vi "PH_TKTDS-30xx.ProcCases.vi"(0 "i ref in":refnum<vi>, 1 "selector":string, 2 "Data":T1, 3 "call cluster":T2={"Object"="", "Selector"="", "CallType"=enum."synchronous", "Async Object"="", "Async Selector"="", "Data Descriptor"="", "Data"=[], "Error #"=0, "Expire"=0}, 5 "error in (no error)":errorcluster) -> (14 "i ref out":refnum<vi>, 17 "answer cluster":T2={"Object"="", "Selector"="", "CallType"=enum."synchronous", "Async Object"="", "Async Selector"="", "Data Descriptor"="", "Data"=[], "Error #"=0, "Expire"=0}, 19 "error out":errorcluster)   [LabVIEW 2014, in "PH_TKTDS-30xx.lvlib"]
doc: "This method is called by a process from within the default case in the event loop. The methods of a class that are linked to events will be called from THIS method. Add your code here."
uses:
  PH_TKTDS-30xx.lvlib
  CS_Core/CSSystem/CoreDefs/CoreDefs.call_type.ctl
  CS_Core/BaseProcess/BaseProcess.descriptor string definition.ctl
  CS_Core/CSSystem/CoreDefs/CoreDefs.rawDataType.ctl
  PH_TKTDS-30xx.Channel Config.ctl
  PH_TKTDS-30xx.Acquisition Config.ctl
  PH_TKTDS-30xx.Trigger Config.ctl
  PH_TKTDS-30xx.Waveform to fetch.ctl
  CS_Core/CSSystem/CoreLib/CoreLib.string 2 byte array.vi
  CS_Core/CSSystem/CoreLib/CoreLib.byte array 2 short.vi
  CS_Core/CSSystem/CoreLib/CoreLib.byte array 2 int.vi
  CS_Core/CSSystem/CoreLib/CoreLib.byte array 2 string.vi
  CS_Core/CSSystem/CoreLib/CoreLib.byte array 2 double.vi
  CS_Core/BaseProcess/BaseProcess.lvlib
  CS_Core/CSSystem/CoreLib/CoreLib.lvlib
  PH_Basics/PH_PSDBWriter/PH_PSDBWriter.lvlib
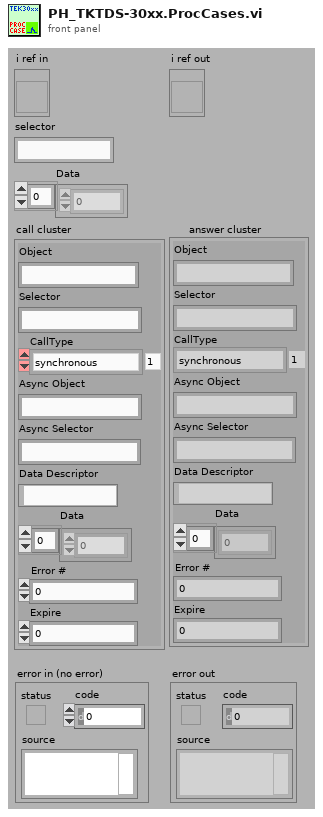
[diagram p1: front panel]
types:
  T1 = typedef "CoreDefs.rawDataType.ctl" = i8[]
  T2 = typedef "CoreDefs.call_type.ctl" = cluster{"Object":string, "Selector":string, "CallType":enum16{"simple", "synchronous", "asynchronous"}, "Async Object":string, "Async Selector":string, "Data Descriptor":T3, "Data":T1, "Error #":i32, "Expire":u32}
  T3 = typedef "BaseProcess.lvlib/BaseProcess.descriptor string definition.ctl" = string
  T4 = typedef "PH_TKTDS-30xx.lvlib/PH_TKTDS-30xx.Channel Config.ctl" = cluster{"Channel Name":string, "Input Impedance":string, "Max Input Frequency":string, "Vertical Coupling":i32, "Channel Enabled":bool, "Probe Attenuation":dbl, "Vertical Range":dbl, "Vertical Offset":dbl}
  T5 = typedef "PH_TKTDS-30xx.lvlib/PH_TKTDS-30xx.Acquisition Config.ctl" = cluster{"Time base":dbl, "Record Length":u16, "Start Time":dbl, "Type":i32, "Continuous":bool}
  T6 = typedef "PH_TKTDS-30xx.lvlib/PH_TKTDS-30xx.Trigger Config.ctl" = cluster{"Source":string, "Slope":i32, "Level [V]":dbl}
  T7 = typedef "PH_TKTDS-30xx.lvlib/PH_TKTDS-30xx.Waveform to fetch.ctl" = cluster{"Source":string, "Waveform Start":i32, "Waveform End":i32}
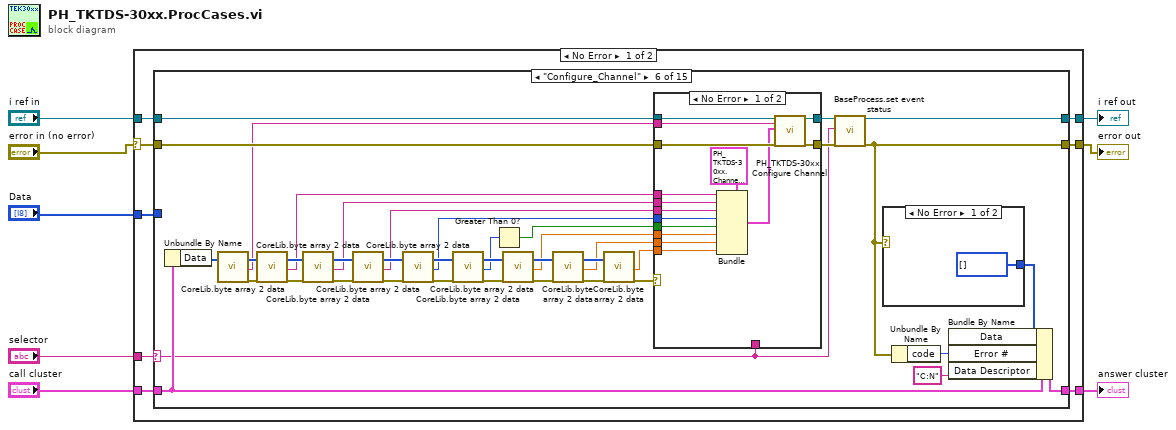
[diagram p0: block diagram]
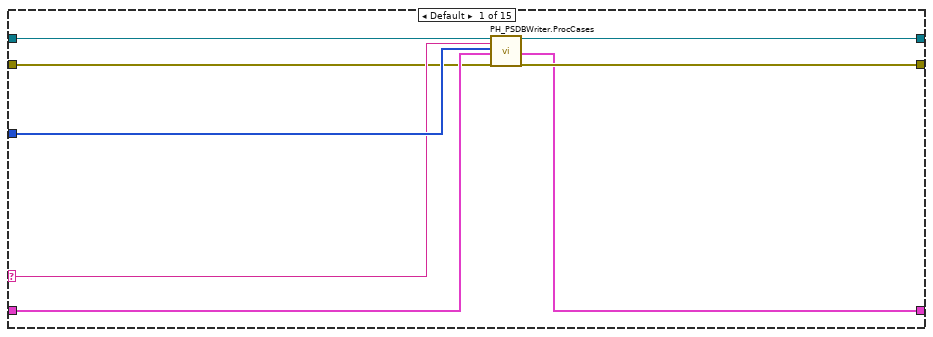
[diagram p2: hidden frame]
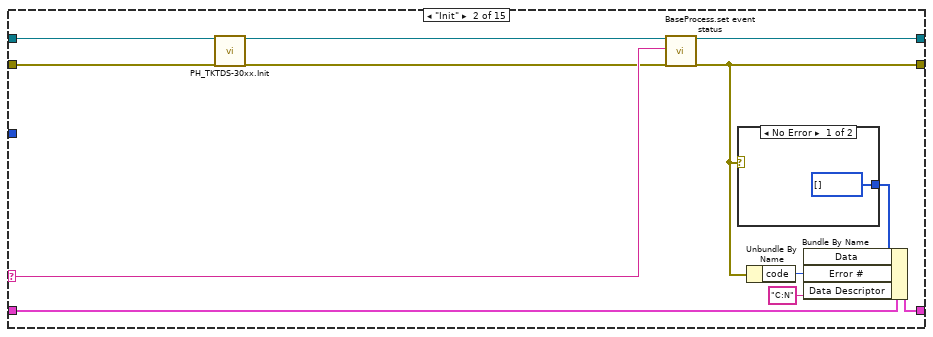
[diagram p3: hidden frame]
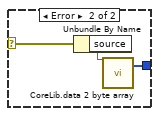
[diagram p4: hidden frame]
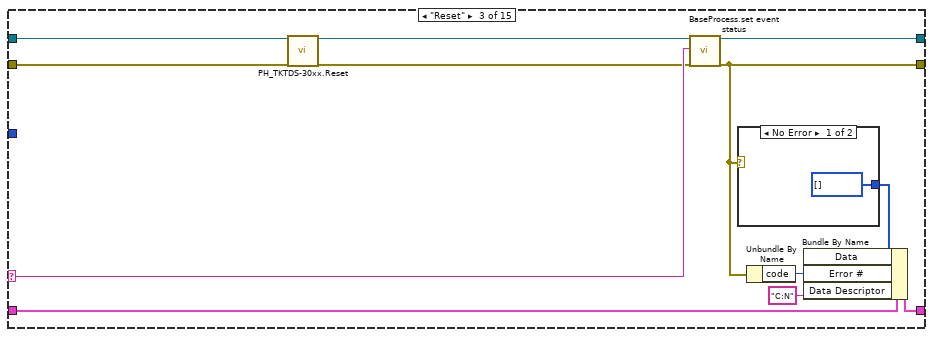
[diagram p5: hidden frame]
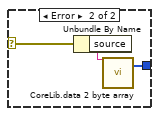
[diagram p6: hidden frame]
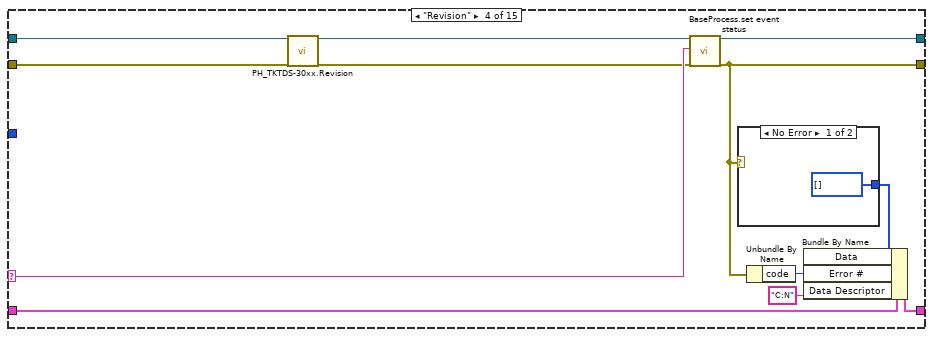
[diagram p7: hidden frame]
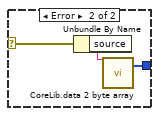
[diagram p8: hidden frame]
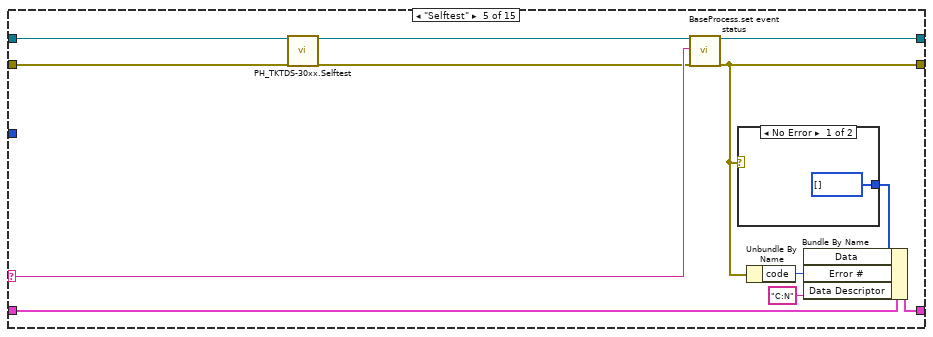
[diagram p9: hidden frame]
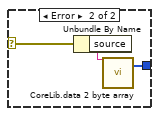
[diagram p10: hidden frame]
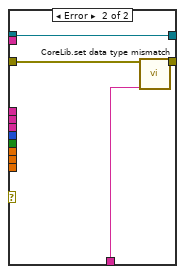
[diagram p11: hidden frame]
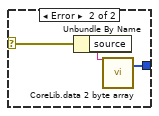
[diagram p12: hidden frame]
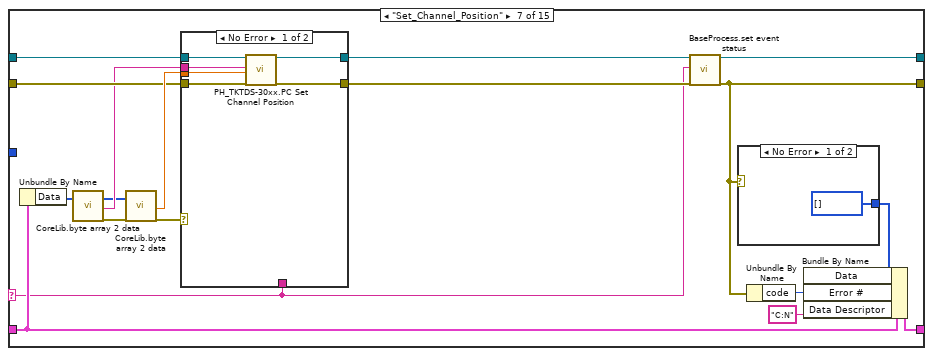
[diagram p13: hidden frame]
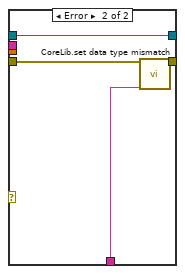
[diagram p14: hidden frame]
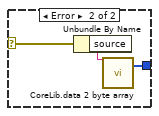
[diagram p15: hidden frame]
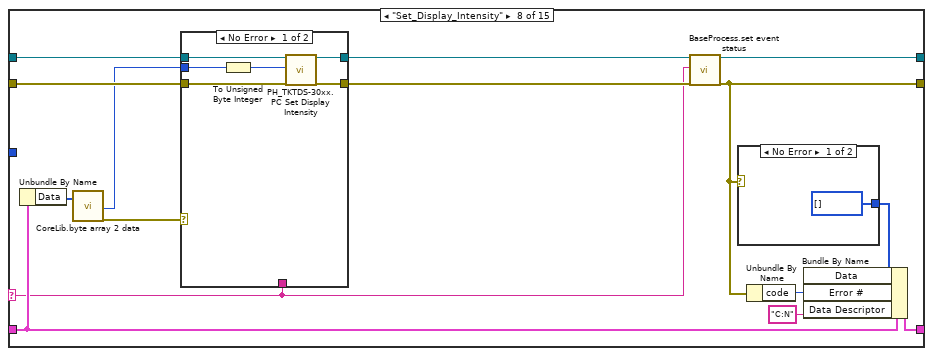
[diagram p16: hidden frame]
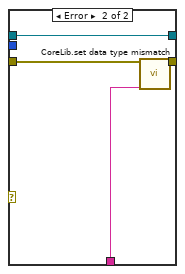
[diagram p17: hidden frame]
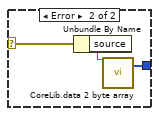
[diagram p18: hidden frame]
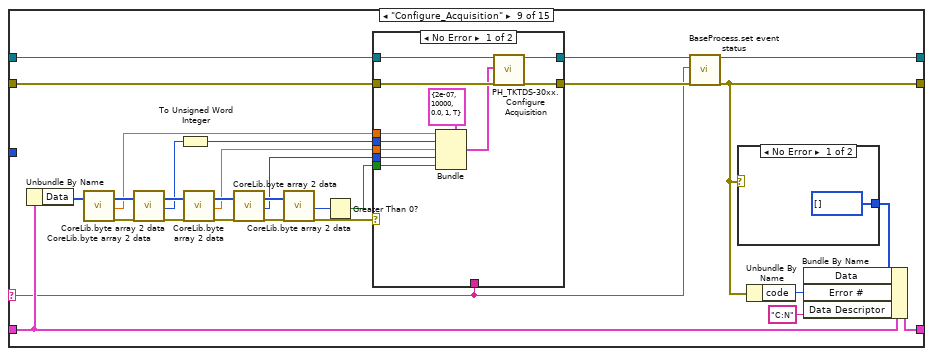
[diagram p19: hidden frame]
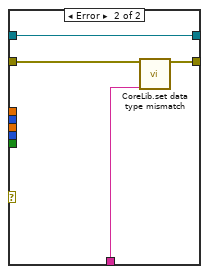
[diagram p20: hidden frame]
diagram:
  n1 = case shown="No Error" "error in (no error)" {
    selector: "error in (no error)" -> [w9 w414]
    tunnel: "selector" -> [w16 _]
    tunnel: [w15 w415] -> w7
    tunnel: "Data" -> [w14 _]
    tunnel: "call cluster" -> [w13 w415]
    tunnel: "i ref in" -> [w12 w416]
    tunnel: [w11 w416] -> w3
    tunnel: [w10 w414] -> w2
    frame No Error {
      n2 = case shown="\"Configure_Channel\"" w16 {
        selector: w16 -> [w19 w29 w45 w61 w77 w98 w158 w188 w219 w263 w301 w337 w367 w386 w402]
        tunnel: w14 -> [w20 _ _ _ _ _ _ _ _ _ _ _ _ _ _]
        tunnel: w12 -> [w18 w28 w44 w60 w76 w122 w163 w192 w235 w275 w313 w343 w371 w385 w401]
        tunnel: [w24 w32 w48 w64 w80 w124 w165 w194 w237 w277 w315 w348 w373 w389 w405] -> w11
        tunnel: w13 -> [w21 w30 w46 w62 w78 w119 w160 w189 w231 w271 w309 w341 w368 w387 w403]
        tunnel: [w22 w35 w51 w67 w83 w127 w168 w197 w240 w280 w318 w351 w376 w392 w408] -> w15
        tunnel: w9 -> [w17 w26 w43 w59 w75 w96 w157 w187 w218 w262 w300 w340 w366 w383 w399]
        tunnel: [w23 w33 w49 w65 w81 w125 w166 w195 w238 w278 w316 w349 w374 w390 w406] -> w10
        frame Default {
          n3 = call "PH_PSDBWriter.ProcCases.vi"("i ref in"=w18, "selector"=w19, "Data"=w20, "call cluster"=w21, "error in"=w17) -> ("i ref out"=w24:refnum<vi>, "answer cluster"=w22:T2, "error out"=w23:errorcluster)  [unwired: 12 in]
        }
        frame "Init" {
          n4 = call "PH_TKTDS-30xx.Init.vi"("i ref in"=w28, "error in (no error)"=w26) -> ("i ref out"=w27:refnum<vi>, "error out"=w25:errorcluster)  [unwired: 16 in]
          n5 = call "BaseProcess.set event status.vi"("i ref in"=w27, "EventStatus"=w29, "error in (no error)"=w25) -> ("i ref out"=w32:refnum<vi>, "error out"=w33:errorcluster)  [unwired: 14 in, 1 out]
          n6 = case shown="No Error" w33 {
            selector: w33 -> [_ w40]
            tunnel: [T1 [] ("byteArray out") w39] -> w34
            frame No Error {
            }
            frame Error {
              n7 = Unbundle By Name(w40) -> ("source"=w38:string)
              n8 = call-poly "CoreLib.data 2 byte array.vi"("string"=w38) -> ("byteArray out"=w39:T1)  [unwired: 18 in]
            }
          }
          n9 = Unbundle By Name(w33) -> ("code"=w36:i32)
          n10 = Bundle By Name(cluster=w30, "Data"=w34, "Error #"=w36, "Data Descriptor"="C:N") -> (w35:T2)
        }
        frame "Reset" {
          n11 = call "PH_TKTDS-30xx.Reset.vi"("i ref in"=w44, "error IO"=w43) -> ("i ref out"=w41:refnum<vi>, "error out"=w42:errorcluster)  [unwired: 16 in]
          n12 = call "BaseProcess.set event status.vi"("i ref in"=w41, "EventStatus"=w45, "error in (no error)"=w42) -> ("i ref out"=w48:refnum<vi>, "error out"=w49:errorcluster)  [unwired: 14 in, 1 out]
          n13 = case shown="No Error" w49 {
            selector: w49 -> [_ w56]
            tunnel: [T1 [] ("byteArray out") w55] -> w50
            frame No Error {
            }
            frame Error {
              n14 = Unbundle By Name(w56) -> ("source"=w54:string)
              n15 = call-poly "CoreLib.data 2 byte array.vi"("string"=w54) -> ("byteArray out"=w55:T1)  [unwired: 18 in]
            }
          }
          n16 = Unbundle By Name(w49) -> ("code"=w52:i32)
          n17 = Bundle By Name(cluster=w46, "Data"=w50, "Error #"=w52, "Data Descriptor"="C:N") -> (w51:T2)
        }
        frame "Revision" {
          n18 = call "PH_TKTDS-30xx.Revision.vi"("i ref in"=w60, "error IO"=w59) -> ("i ref out"=w57:refnum<vi>, "error out"=w58:errorcluster)  [unwired: 16 in]
          n19 = call "BaseProcess.set event status.vi"("i ref in"=w57, "EventStatus"=w61, "error in (no error)"=w58) -> ("i ref out"=w64:refnum<vi>, "error out"=w65:errorcluster)  [unwired: 14 in, 1 out]
          n20 = case shown="No Error" w65 {
            selector: w65 -> [_ w72]
            tunnel: [T1 [] ("byteArray out") w71] -> w66
            frame No Error {
            }
            frame Error {
              n21 = Unbundle By Name(w72) -> ("source"=w70:string)
              n22 = call-poly "CoreLib.data 2 byte array.vi"("string"=w70) -> ("byteArray out"=w71:T1)  [unwired: 18 in]
            }
          }
          n23 = Unbundle By Name(w65) -> ("code"=w68:i32)
          n24 = Bundle By Name(cluster=w62, "Data"=w66, "Error #"=w68, "Data Descriptor"="C:N") -> (w67:T2)
        }
        frame "Selftest" {
          n25 = call "PH_TKTDS-30xx.Selftest.vi"("i ref in"=w76, "error IO"=w75) -> ("i ref out"=w73:refnum<vi>, "error out"=w74:errorcluster)  [unwired: 16 in]
          n26 = call "BaseProcess.set event status.vi"("i ref in"=w73, "EventStatus"=w77, "error in (no error)"=w74) -> ("i ref out"=w80:refnum<vi>, "error out"=w81:errorcluster)  [unwired: 14 in, 1 out]
          n27 = case shown="No Error" w81 {
            selector: w81 -> [_ w88]
            tunnel: [T1 [] ("byteArray out") w87] -> w82
            frame No Error {
            }
            frame Error {
              n28 = Unbundle By Name(w88) -> ("source"=w86:string)
              n29 = call-poly "CoreLib.data 2 byte array.vi"("string"=w86) -> ("byteArray out"=w87:T1)  [unwired: 18 in]
            }
          }
          n30 = Unbundle By Name(w81) -> ("code"=w84:i32)
          n31 = Bundle By Name(cluster=w78, "Data"=w82, "Error #"=w84, "Data Descriptor"="C:N") -> (w83:T2)
        }
        frame "Configure_Channel" {
          n32 = Unbundle By Name(w119) -> ("Data"=w92:T1)
          n33 = call-poly "CoreLib.byte array 2 data.vi"("byteArray"=w92) -> ("byteArray out"=w91:T1, "string"=w89:string, "error out"=w90:errorcluster)  [unwired: 16 in]
          n34 = call-poly "CoreLib.byte array 2 data.vi"("byteArray"=w91, "error in (no error)"=w90) -> ("byteArray out"=w111:T1, "string"=w104:string, "error out"=w118:errorcluster)  [unwired: 15 in]
          n35 = call-poly "CoreLib.byte array 2 data.vi"("byteArray"=w111, "error in (no error)"=w118) -> ("byteArray out"=w110:T1, "string"=w103:string, "error out"=w117:errorcluster)  [unwired: 15 in]
          n36 = call-poly "CoreLib.byte array 2 data.vi"("byteArray"=w110, "error in (no error)"=w117) -> ("byteArray out"=w109:T1, "string"=w102:string, "error out"=w116:errorcluster)  [unwired: 15 in]
          n37 = call-poly "CoreLib.byte array 2 data.vi"("byteArray"=w109, "error in (no error)"=w116) -> ("byteArray out"=w108:T1, "i32"=w93:i32, "error out"=w115:errorcluster)  [unwired: 15 in]
          n38 = call-poly "CoreLib.byte array 2 data.vi"("byteArray"=w108, "error in (no error)"=w115) -> ("byteArray out"=w107:T1, "i16"=w95:i16, "error out"=w114:errorcluster)  [unwired: 15 in]
          n39 = Greater Than 0?(x=w95) -> (x > 0?=w94:bool)
          n40 = call-poly "CoreLib.byte array 2 data.vi"("byteArray"=w107, "error in (no error)"=w114) -> ("byteArray out"=w106:T1, "d64"=w101:dbl, "error out"=w113:errorcluster)  [unwired: 15 in]
          n41 = call-poly "CoreLib.byte array 2 data.vi"("byteArray"=w106, "error in (no error)"=w113) -> ("byteArray out"=w105:T1, "d64"=w100:dbl, "error out"=w112:errorcluster)  [unwired: 15 in]
          n42 = call-poly "CoreLib.byte array 2 data.vi"("byteArray"=w105, "error in (no error)"=w112) -> ("d64"=w99:dbl, "error out"=w97:errorcluster)  [unwired: 15 in, 1 out]
          n43 = case shown="No Error" w97 {
            tunnel: w122 -> [w143 w147]
            tunnel: [w142 w145] -> w121
            tunnel: [w141 w147] -> w120
            tunnel: w104 -> [w139 _]
            tunnel: w103 -> [w138 _]
            tunnel: w102 -> [w137 _]
            tunnel: w93 -> [w136 _]
            tunnel: w94 -> [w135 _]
            tunnel: w101 -> [w134 _]
            tunnel: w100 -> [w133 _]
            tunnel: w99 -> [w132 _]
            tunnel: w98 -> [_ w146]
            tunnel: w96 -> [w140 w144]
            tunnel: w89 -> [w130 _]
            frame No Error {
              n44 = Bundle(cluster=T4 {"Channel Name"="CH1", "Input Impedance"="MEG", "Max Input Frequency"="TWENTY", "Vertical Coupling"=1, "Channel Enabled"=TRUE, "Probe Attenuation"=1.0, "Vertical Range"=100.0, "Vertical Offset"=0.0} ("Channel Config 2"), "Channel Name"=w139, "Input Impedance"=w138, "Max Input Frequency"=w137, "Vertical Coupling"=w136, "Channel Enabled"=w135, "Probe Attenuation"=w134, "Vertical Range"=w133, "Vertical Offset"=w132) -> (w131:T4)
              n45 = call "PH_TKTDS-30xx.Configure Channel.vi"("i ref in"=w143, "GUI Element Name"=w130, "Channel Configuration"=w131, "error IO"=w140) -> ("i ref out"=w141:refnum<vi>, "error out"=w142:errorcluster)  [unwired: 14 in]
            }
            frame Error {
              n46 = call "CoreLib.set data type mismatch.vi"("error in (no error)"=w144, "error source"=w146) -> ("error out"=w145:errorcluster)  [unwired: 17 in]
            }
          }
          n47 = call "BaseProcess.set event status.vi"("i ref in"=w120, "EventStatus"=w98, "error in (no error)"=w121) -> ("i ref out"=w124:refnum<vi>, "error out"=w125:errorcluster)  [unwired: 14 in, 1 out]
          n48 = case shown="No Error" w125 {
            selector: w125 -> [_ w151]
            tunnel: [T1 [] ("byteArray out") w150] -> w126
            frame No Error {
            }
            frame Error {
              n49 = Unbundle By Name(w151) -> ("source"=w149:string)
              n50 = call-poly "CoreLib.data 2 byte array.vi"("string"=w149) -> ("byteArray out"=w150:T1)  [unwired: 18 in]
            }
          }
          n51 = Unbundle By Name(w125) -> ("code"=w128:i32)
          n52 = Bundle By Name(cluster=w119, "Data"=w126, "Error #"=w128, "Data Descriptor"="C:N") -> (w127:T2)
        }
        frame "Set_Channel_Position" {
          n53 = Unbundle By Name(w160) -> ("Data"=w156:T1)
          n54 = call-poly "CoreLib.byte array 2 data.vi"("byteArray"=w156) -> ("byteArray out"=w153:T1, "string"=w155:string, "error out"=w154:errorcluster)  [unwired: 16 in]
          n55 = call-poly "CoreLib.byte array 2 data.vi"("byteArray"=w153, "error in (no error)"=w154) -> ("d64"=w159:dbl, "error out"=w152:errorcluster)  [unwired: 15 in, 1 out]
          n56 = case shown="No Error" w152 {
            tunnel: w163 -> [w175 w179]
            tunnel: [w174 w177] -> w162
            tunnel: [w173 w179] -> w161
            tunnel: w159 -> [w170 _]
            tunnel: w158 -> [_ w178]
            tunnel: w157 -> [w172 w176]
            tunnel: w155 -> [w171 _]
            frame No Error {
              n57 = call "PH_TKTDS-30xx.PC Set Channel Position.vi"("i ref in"=w175, "Channel Name"=w171, "Position (0)"=w170, "error IO"=w172) -> ("i ref out"=w173:refnum<vi>, "error out"=w174:errorcluster)  [unwired: 14 in]
            }
            frame Error {
              n58 = call "CoreLib.set data type mismatch.vi"("error in (no error)"=w176, "error source"=w178) -> ("error out"=w177:errorcluster)  [unwired: 17 in]
            }
          }
          n59 = call "BaseProcess.set event status.vi"("i ref in"=w161, "EventStatus"=w158, "error in (no error)"=w162) -> ("i ref out"=w165:refnum<vi>, "error out"=w166:errorcluster)  [unwired: 14 in, 1 out]
          n60 = case shown="No Error" w166 {
            selector: w166 -> [_ w183]
            tunnel: [T1 [] ("byteArray out") w182] -> w167
            frame No Error {
            }
            frame Error {
              n61 = Unbundle By Name(w183) -> ("source"=w181:string)
              n62 = call-poly "CoreLib.data 2 byte array.vi"("string"=w181) -> ("byteArray out"=w182:T1)  [unwired: 18 in]
            }
          }
          n63 = Unbundle By Name(w166) -> ("code"=w169:i32)
          n64 = Bundle By Name(cluster=w160, "Data"=w167, "Error #"=w169, "Data Descriptor"="C:N") -> (w168:T2)
        }
        frame "Set_Display_Intensity" {
          n65 = Unbundle By Name(w189) -> ("Data"=w186:T1)
          n66 = call-poly "CoreLib.byte array 2 data.vi"("byteArray"=w186) -> ("i16"=w185:i16, "error out"=w184:errorcluster)  [unwired: 16 in, 1 out]
          n67 = case shown="No Error" w184 {
            tunnel: w192 -> [w204 w208]
            tunnel: [w203 w206] -> w191
            tunnel: [w202 w208] -> w190
            tunnel: w188 -> [_ w207]
            tunnel: w187 -> [w201 w205]
            tunnel: w185 -> [w200 _]
            frame No Error {
              n68 = To Unsigned Byte Integer(number=w200) -> (unsigned 8bit integer=w199:u8)
              n69 = call "PH_TKTDS-30xx.PC Set Display Intensity.vi"("i ref in"=w204, "Intensity (1)"=w199, "error IO"=w201) -> ("i ref out"=w202:refnum<vi>, "error out"=w203:errorcluster)  [unwired: 15 in]
            }
            frame Error {
              n70 = call "CoreLib.set data type mismatch.vi"("error in (no error)"=w205, "error source"=w207) -> ("error out"=w206:errorcluster)  [unwired: 17 in]
            }
          }
          n71 = call "BaseProcess.set event status.vi"("i ref in"=w190, "EventStatus"=w188, "error in (no error)"=w191) -> ("i ref out"=w194:refnum<vi>, "error out"=w195:errorcluster)  [unwired: 14 in, 1 out]
          n72 = case shown="No Error" w195 {
            selector: w195 -> [_ w212]
            tunnel: [T1 [] ("byteArray out") w211] -> w196
            frame No Error {
            }
            frame Error {
              n73 = Unbundle By Name(w212) -> ("source"=w210:string)
              n74 = call-poly "CoreLib.data 2 byte array.vi"("string"=w210) -> ("byteArray out"=w211:T1)  [unwired: 18 in]
            }
          }
          n75 = Unbundle By Name(w195) -> ("code"=w198:i32)
          n76 = Bundle By Name(cluster=w189, "Data"=w196, "Error #"=w198, "Data Descriptor"="C:N") -> (w197:T2)
        }
        frame "Configure_Acquisition" {
          n77 = Unbundle By Name(w231) -> ("Data"=w232:T1)
          n78 = call-poly "CoreLib.byte array 2 data.vi"("byteArray"=w232) -> ("byteArray out"=w226:T1, "d64"=w222:dbl, "error out"=w230:errorcluster)  [unwired: 16 in]
          n79 = call-poly "CoreLib.byte array 2 data.vi"("byteArray"=w226, "error in (no error)"=w230) -> ("byteArray out"=w225:T1, "i16"=w221:i16, "error out"=w229:errorcluster)  [unwired: 15 in]
          n80 = To Unsigned Word Integer(number=w221) -> (unsigned 16bit integer=w214:u16)
          n81 = call-poly "CoreLib.byte array 2 data.vi"("byteArray"=w225, "error in (no error)"=w229) -> ("byteArray out"=w224:T1, "d64"=w220:dbl, "error out"=w228:errorcluster)  [unwired: 15 in]
          n82 = call-poly "CoreLib.byte array 2 data.vi"("byteArray"=w224, "error in (no error)"=w228) -> ("byteArray out"=w223:T1, "i32"=w215:i32, "error out"=w227:errorcluster)  [unwired: 15 in]
          n83 = call-poly "CoreLib.byte array 2 data.vi"("byteArray"=w223, "error in (no error)"=w227) -> ("i16"=w217:i16, "error out"=w213:errorcluster)  [unwired: 15 in, 1 out]
          n84 = Greater Than 0?(x=w217) -> (x > 0?=w216:bool)
          n85 = case shown="No Error" w213 {
            tunnel: w235 -> [w252 w256]
            tunnel: [w251 w254] -> w234
            tunnel: [w250 w256] -> w233
            tunnel: w222 -> [w248 _]
            tunnel: w214 -> [w247 _]
            tunnel: w220 -> [w246 _]
            tunnel: w215 -> [w245 _]
            tunnel: w216 -> [w244 _]
            tunnel: w219 -> [_ w255]
            tunnel: w218 -> [w249 w253]
            frame No Error {
              n86 = Bundle(cluster=T5 {"Time base"=2e-07, "Record Length"=10000, "Start Time"=0.0, "Type"=1, "Continuous"=TRUE} ("Acqu Config 2"), "Time base"=w248, "Record Length"=w247, "Start Time"=w246, "Type"=w245, "Continuous"=w244) -> (w243:T5)
              n87 = call "PH_TKTDS-30xx.Configure Acquisition.vi"("i ref in"=w252, "Acquisition Configuration"=w243, "error IO"=w249) -> ("i ref out"=w250:refnum<vi>, "error out"=w251:errorcluster)  [unwired: 15 in]
            }
            frame Error {
              n88 = call "CoreLib.set data type mismatch.vi"("error in (no error)"=w253, "error source"=w255) -> ("error out"=w254:errorcluster)  [unwired: 17 in]
            }
          }
          n89 = call "BaseProcess.set event status.vi"("i ref in"=w233, "EventStatus"=w219, "error in (no error)"=w234) -> ("i ref out"=w237:refnum<vi>, "error out"=w238:errorcluster)  [unwired: 14 in, 1 out]
          n90 = case shown="No Error" w238 {
            selector: w238 -> [_ w260]
            tunnel: [T1 [] ("byteArray out") w259] -> w239
            frame No Error {
            }
            frame Error {
              n91 = Unbundle By Name(w260) -> ("source"=w258:string)
              n92 = call-poly "CoreLib.data 2 byte array.vi"("string"=w258) -> ("byteArray out"=w259:T1)  [unwired: 18 in]
            }
          }
          n93 = Unbundle By Name(w238) -> ("code"=w241:i32)
          n94 = Bundle By Name(cluster=w231, "Data"=w239, "Error #"=w241, "Data Descriptor"="C:N") -> (w240:T2)
        }
        frame "Configure_Trigger" {
          n95 = Unbundle By Name(w271) -> ("Data"=w272:T1)
          n96 = call-poly "CoreLib.byte array 2 data.vi"("byteArray"=w272) -> ("byteArray out"=w268:T1, "string"=w266:string, "error out"=w270:errorcluster)  [unwired: 16 in]
          n97 = call-poly "CoreLib.byte array 2 data.vi"("byteArray"=w268, "error in (no error)"=w270) -> ("byteArray out"=w267:T1, "i32"=w265:i32, "error out"=w269:errorcluster)  [unwired: 15 in]
          n98 = call-poly "CoreLib.byte array 2 data.vi"("byteArray"=w267, "error in (no error)"=w269) -> ("d64"=w264:dbl, "error out"=w261:errorcluster)  [unwired: 15 in, 1 out]
          n99 = case shown="No Error" w261 {
            tunnel: w275 -> [w290 w294]
            tunnel: [w289 w292] -> w274
            tunnel: [w288 w294] -> w273
            tunnel: w266 -> [w285 _]
            tunnel: w265 -> [w284 _]
            tunnel: w264 -> [w283 _]
            tunnel: w263 -> [_ w293]
            tunnel: w262 -> [w287 w291]
            frame No Error {
              n100 = Bundle(cluster=T6 {"Source"="CH1", "Slope"=0, "Level [V]"=0.0} ("Trig Config"), "Source"=w285, "Slope"=w284, "Level [V]"=w283) -> (w282:T6)
              n101 = call "PH_TKTDS-30xx.Configure Trigger.vi"("i ref in"=w290, "Trigger Configuration"=w282, "error IO"=w287) -> ("i ref out"=w288:refnum<vi>, "error out"=w289:errorcluster)  [unwired: 15 in]
            }
            frame Error {
              n102 = call "CoreLib.set data type mismatch.vi"("error in (no error)"=w291, "error source"=w293) -> ("error out"=w292:errorcluster)  [unwired: 17 in]
            }
          }
          n103 = call "BaseProcess.set event status.vi"("i ref in"=w273, "EventStatus"=w263, "error in (no error)"=w274) -> ("i ref out"=w277:refnum<vi>, "error out"=w278:errorcluster)  [unwired: 14 in, 1 out]
          n104 = case shown="No Error" w278 {
            selector: w278 -> [_ w298]
            tunnel: [T1 [] ("byteArray out") w297] -> w279
            frame No Error {
            }
            frame Error {
              n105 = Unbundle By Name(w298) -> ("source"=w296:string)
              n106 = call-poly "CoreLib.data 2 byte array.vi"("string"=w296) -> ("byteArray out"=w297:T1)  [unwired: 18 in]
            }
          }
          n107 = Unbundle By Name(w278) -> ("code"=w281:i32)
          n108 = Bundle By Name(cluster=w271, "Data"=w279, "Error #"=w281, "Data Descriptor"="C:N") -> (w280:T2)
        }
        frame "Fetch_Waveform" {
          n109 = Unbundle By Name(w309) -> ("Data"=w310:T1)
          n110 = call-poly "CoreLib.byte array 2 data.vi"("byteArray"=w310) -> ("byteArray out"=w306:T1, "string"=w304:string, "error out"=w308:errorcluster)  [unwired: 16 in]
          n111 = call-poly "CoreLib.byte array 2 data.vi"("byteArray"=w306, "error in (no error)"=w308) -> ("byteArray out"=w305:T1, "i32"=w303:i32, "error out"=w307:errorcluster)  [unwired: 15 in]
          n112 = call-poly "CoreLib.byte array 2 data.vi"("byteArray"=w305, "error in (no error)"=w307) -> ("i32"=w302:i32, "error out"=w299:errorcluster)  [unwired: 15 in, 1 out]
          n113 = case shown="No Error" w299 {
            tunnel: w313 -> [w328 w332]
            tunnel: [w327 w330] -> w312
            tunnel: [w326 w332] -> w311
            tunnel: w304 -> [w324 _]
            tunnel: w303 -> [w323 _]
            tunnel: w302 -> [w322 _]
            tunnel: w301 -> [_ w331]
            tunnel: w300 -> [w325 w329]
            frame No Error {
              n114 = Bundle(cluster=T7 {"Source"="CH1", "Waveform Start"=0, "Waveform End"=0} ("Wave 2 fetch 2"), "Source"=w324, "Waveform Start"=w323, "Waveform End"=w322) -> (w321:T7)
              n115 = call "PH_TKTDS-30xx.Fetch Waveform.vi"("i ref in"=w328, "Waveform to fetch"=w321, "error IO"=w325) -> ("i ref out"=w326:refnum<vi>, "error out"=w327:errorcluster)  [unwired: 15 in]
            }
            frame Error {
              n116 = call "CoreLib.set data type mismatch.vi"("error in (no error)"=w329, "error source"=w331) -> ("error out"=w330:errorcluster)  [unwired: 17 in]
            }
          }
          n117 = call "BaseProcess.set event status.vi"("i ref in"=w311, "EventStatus"=w301, "error in (no error)"=w312) -> ("i ref out"=w315:refnum<vi>, "error out"=w316:errorcluster)  [unwired: 14 in, 1 out]
          n118 = case shown="No Error" w316 {
            selector: w316 -> [_ w336]
            tunnel: [T1 [] ("byteArray out") w335] -> w317
            frame No Error {
            }
            frame Error {
              n119 = Unbundle By Name(w336) -> ("source"=w334:string)
              n120 = call-poly "CoreLib.data 2 byte array.vi"("string"=w334) -> ("byteArray out"=w335:T1)  [unwired: 18 in]
            }
          }
          n121 = Unbundle By Name(w316) -> ("code"=w319:i32)
          n122 = Bundle By Name(cluster=w309, "Data"=w317, "Error #"=w319, "Data Descriptor"="C:N") -> (w318:T2)
        }
        frame "Remote Control" {
          n123 = Unbundle By Name(w341) -> ("Data"=w345:T1)
          n124 = call-poly "CoreLib.byte array 2 data.vi"("byteArray"=w345) -> ("i16"=w346:i16, "error out"=w344:errorcluster)  [unwired: 16 in, 1 out]
          n125 = Greater Than 0?(x=w346) -> (x > 0?=w338:bool)
          n126 = case shown="No Error" w344 {
            tunnel: [w354 w361] -> w342
            tunnel: w343 -> [w356 w361]
            tunnel: w340 -> [w355 w360]
            tunnel: [w357 w359] -> w339
            tunnel: w337 -> [_ w358]
            tunnel: w338 -> [w353 _]
            frame No Error {
              n127 = call "PH_TKTDS-30xx.PC Set Remote Control.vi"("i ref in"=w356, "Remote Controlled?"=w353, "error in (no error)"=w355) -> ("i ref out"=w354:refnum<vi>, "error out"=w357:errorcluster)  [unwired: 15 in]
            }
            frame Error {
              n128 = call "CoreLib.set data type mismatch.vi"("error in (no error)"=w360, "error source"=w358) -> ("error out"=w359:errorcluster)  [unwired: 17 in]
            }
          }
          n129 = call "BaseProcess.set event status.vi"("i ref in"=w342, "EventStatus"=w337, "error in (no error)"=w339) -> ("i ref out"=w348:refnum<vi>, "error out"=w349:errorcluster)  [unwired: 14 in, 1 out]
          n130 = case shown="No Error" w349 {
            selector: w349 -> [_ w365]
            tunnel: [T1 [] ("byteArray out") w364] -> w350
            frame No Error {
            }
            frame Error {
              n131 = Unbundle By Name(w365) -> ("source"=w363:string)
              n132 = call-poly "CoreLib.data 2 byte array.vi"("string"=w363) -> ("byteArray out"=w364:T1)  [unwired: 18 in]
            }
          }
          n133 = Unbundle By Name(w349) -> ("code"=w352:i32)
          n134 = Bundle By Name(cluster=w341, "Data"=w350, "Error #"=w352, "Data Descriptor"="C:N") -> (w351:T2)
        }
        frame "Clear" {
          n135 = call "PH_TKTDS-30xx.Clear.vi"("i ref in"=w371, "error IO"=w366) -> ("i ref out"=w369:refnum<vi>, "error out"=w370:errorcluster)  [unwired: 16 in]
          n136 = call "BaseProcess.set event status.vi"("i ref in"=w369, "EventStatus"=w367, "error in (no error)"=w370) -> ("i ref out"=w373:refnum<vi>, "error out"=w374:errorcluster)  [unwired: 14 in, 1 out]
          n137 = case shown="No Error" w374 {
            selector: w374 -> [_ w381]
            tunnel: [T1 [] ("byteArray out") w380] -> w375
            frame No Error {
            }
            frame Error {
              n138 = Unbundle By Name(w381) -> ("source"=w379:string)
              n139 = call-poly "CoreLib.data 2 byte array.vi"("string"=w379) -> ("byteArray out"=w380:T1)  [unwired: 18 in]
            }
          }
          n140 = Unbundle By Name(w374) -> ("code"=w377:i32)
          n141 = Bundle By Name(cluster=w368, "Data"=w375, "Error #"=w377, "Data Descriptor"="C:N") -> (w376:T2)
        }
        frame "Close" {
          n142 = call "PH_TKTDS-30xx.Close.vi"("i ref in"=w385, "error in(no error)"=w383) -> ("i ref out"=w384:refnum<vi>, "error out"=w382:errorcluster)  [unwired: 16 in]
          n143 = call "BaseProcess.set event status.vi"("i ref in"=w384, "EventStatus"=w386, "error in (no error)"=w382) -> ("i ref out"=w389:refnum<vi>, "error out"=w390:errorcluster)  [unwired: 14 in, 1 out]
          n144 = case shown="No Error" w390 {
            selector: w390 -> [_ w397]
            tunnel: [T1 [] ("byteArray out") w396] -> w391
            frame No Error {
            }
            frame Error {
              n145 = Unbundle By Name(w397) -> ("source"=w395:string)
              n146 = call-poly "CoreLib.data 2 byte array.vi"("string"=w395) -> ("byteArray out"=w396:T1)  [unwired: 18 in]
            }
          }
          n147 = Unbundle By Name(w390) -> ("code"=w393:i32)
          n148 = Bundle By Name(cluster=w387, "Data"=w391, "Error #"=w393, "Data Descriptor"="C:N") -> (w392:T2)
        }
        frame "Set_Bin_Data_Encoding" {
          n149 = call "PH_TKTDS-30xx.Set Bin Data Encoding.vi"("i ref in"=w401, "error IO"=w399) -> ("i ref out"=w400:refnum<vi>, "error out"=w398:errorcluster)  [unwired: 16 in]
          n150 = call "BaseProcess.set event status.vi"("i ref in"=w400, "EventStatus"=w402, "error in (no error)"=w398) -> ("i ref out"=w405:refnum<vi>, "error out"=w406:errorcluster)  [unwired: 14 in, 1 out]
          n151 = case shown="No Error" w406 {
            selector: w406 -> [_ w413]
            tunnel: [T1 [] ("byteArray out") w412] -> w407
            frame No Error {
            }
            frame Error {
              n152 = Unbundle By Name(w413) -> ("source"=w411:string)
              n153 = call-poly "CoreLib.data 2 byte array.vi"("string"=w411) -> ("byteArray out"=w412:T1)  [unwired: 18 in]
            }
          }
          n154 = Unbundle By Name(w406) -> ("code"=w409:i32)
          n155 = Bundle By Name(cluster=w403, "Data"=w407, "Error #"=w409, "Data Descriptor"="C:N") -> (w408:T2)
        }
      }
    }
    frame Error {
    }
  }
  "answer cluster" <- w7
  "i ref out" <- w3
  "error out" <- w2
